vi "Get Interface Info.vi"(8 "error in (no error)":errorcluster, 11 "Device Item Ref in":T1 format="%.0x") -> (0 "error out":errorcluster, 1 "Unit ID":u16, 2 "Name":string, 3 "Item Ref out":T1 format="%.0x", 4 "Refresh Rate":i32, 5 "Interface Type":T2)   [LabVIEW 2021, in "Modbus Master System Explorer.lvlib"]
uses:
  Modbus Master System Explorer.lvlib
  Shared/Controls/Interface Type.ctl
  <vilib>/NI VeriStand/Custom Device API/Custom Device Item Ref.ctl
  Shared/Constants.vi
  <vilib>/NI VeriStand/Custom Device API/Get Item Property (U16).vi
  <vilib>/NI VeriStand/Custom Device API/Get Item Property (I32).vi
  <vilib>/NI VeriStand/Custom Device API/Custom Device API.lvlib
  Shared/Modbus Master Shared.lvlib
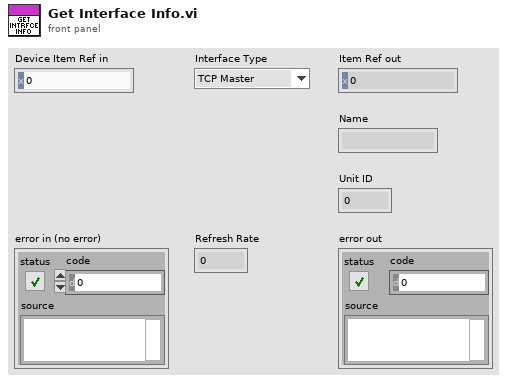
[diagram p1: front panel]
types:
  T1 = typedef "Custom Device API.lvlib/Custom Device Item Ref.ctl" = u64
  T2 = typedef "Modbus Master Shared.lvlib/Interface Type.ctl" = enum16{"TCP Master", "Serial Master", "TCP Slave", "Serial Slave"}
  T3 = typedef "Custom Device API.lvlib/Custom Device Item Info.ctl" = cluster{"Name":string, "Is Channel":bool, "GUID":string, "Is Waveform":bool}
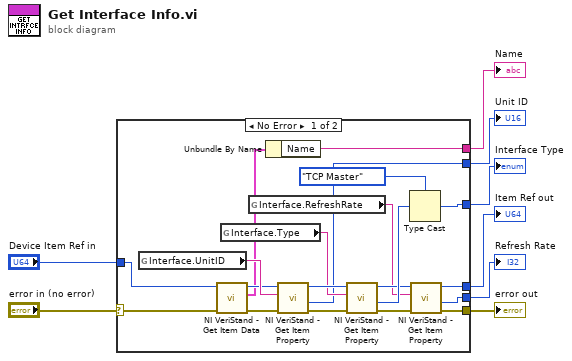
[diagram p0: block diagram]
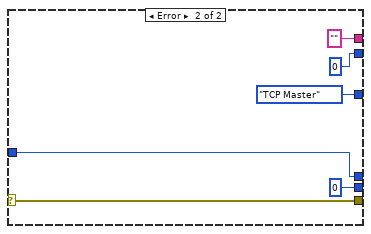
[diagram p2: hidden frame]
diagram:
  n1 = case shown="No Error" "error in (no error)" {
    selector: "error in (no error)" -> [w27 w34]
    tunnel: [w9 w34] -> w8
    tunnel: [w25 Interface_Type."TCP Master" ("Interface Type")] -> w6
    tunnel: [w20 u16 0 ("Value")] -> w5
    tunnel: [w17 "" ("Name")] -> w4
    tunnel: "Device Item Ref in" -> [w15 w33]
    tunnel: [w12 w33] -> w2
    tunnel: [w11 0 ("Value")] -> w1
    frame No Error {
      n2 = global read "Constants.vi" "Interface.UnitID"() -> (w19:string)
      n3 = call <vilib>:"NI VeriStand - Get Item Data.vi"("error in (no error)"=w27, "Item Ref in"=w15) -> ("error out"=w28:errorcluster, "Item Info"=w16:T3, "Item Ref out"=w18:T1)  [unwired: 7 out]
      n4 = global read "Constants.vi" "Interface.Type"() -> (w21:string)
      n5 = global read "Constants.vi" "Interface.RefreshRate"() -> (w13:string)
      n6 = Unbundle By Name(w16) -> ("Name"=w17:string)
      n7 = call-poly <vilib>:"NI VeriStand - Get Item Property.vi"("error in (no error)"=w28, "Property Name"=w19, "Item Ref in"=w18) -> ("error out"=w26:errorcluster, "Value"=w20:u16, "Item Ref out"=w22:T1)  [unwired: 5 in, 1 out]
      n8 = call-poly <vilib>:"NI VeriStand - Get Item Property.vi"("error in (no error)"=w26, "Property Name"=w21, "Item Ref in"=w22) -> ("error out"=w10:errorcluster, "Value"=w24:u16, "Item Ref out"=w14:T1)  [unwired: 5 in, 1 out]
      n9 = Type Cast(type=Interface_Type."TCP Master" ("Interface Type"), x=w24) -> (*(type *) &x=w25:T2)
      n10 = call-poly <vilib>:"NI VeriStand - Get Item Property.vi"("error in (no error)"=w10, "Property Name"=w13, "Item Ref in"=w14) -> ("error out"=w9:errorcluster, "Value"=w11:i32, "Item Ref out"=w12:T1)  [unwired: 5 in, 1 out]
    }
    frame Error {
    }
  }
  "error out" <- w8
  "Interface Type" <- w6
  "Unit ID" <- w5
  "Name" <- w4
  "Item Ref out" <- w2
  "Refresh Rate" <- w1
